vi "FIFO.vi"   [LabVIEW 2011, in "FIFO.lvlib"]
uses:
  <instrlib>/RF-RIO/FIFO/FIFO/FPGA/FIFO.lvlib
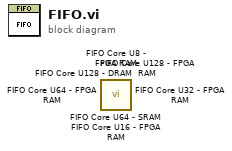
[diagram p0: block diagram]
diagram:
  n1 = call <instrlib>:"FIFO Core U64 - SRAM.vi"() -> ()  [unwired: 12 in, 4 out]
  n2 = call <instrlib>:"FIFO Core U128 - FPGA RAM.vi"() -> ()  [unwired: 12 in, 4 out]
  n3 = call <instrlib>:"FIFO Core U64 - FPGA RAM.vi"() -> ()  [unwired: 12 in, 4 out]
  n4 = call <instrlib>:"FIFO Core U32 - FPGA RAM.vi"() -> ()  [unwired: 12 in, 4 out]
  n5 = call <instrlib>:"FIFO Core U16 - FPGA RAM.vi"() -> ()  [unwired: 12 in, 4 out]
  n6 = call <instrlib>:"FIFO Core U128 - DRAM.vi"() -> ()  [unwired: 12 in, 4 out]
  n7 = call <instrlib>:"FIFO Core U8 - FPGA RAM.vi"() -> ()  [unwired: 12 in, 4 out]
